vi "StageTest2.vi"() -> ()   [LabVIEW 2020]
uses:
  SettingCtrlOptions.ctl
  StageOptions.ctl
  PosCtrlOptions.ctl
  libximc.lvlib
panel:
  in  "Mode":enum16{"Raster", "Serpentine"}(ring)
  in  "Stop":bool
  in  "Y End":sgl=8.0
  in  "Y Start":sgl
  in  "X End":sgl=10.0
  in  "X Start":sgl
  in  "Pixel Count":i32=6
  out "Stage Position":cluster{sgl[], sgl[]}(graph)
  in  "Line Count":i32=6
  out "IDs":i32[](array[numeric])
  out "Calibration":cluster{dbl, "MicrostepMode":u32}[](array[cluster])
  in  "Speed (mm/s)":sgl
  out "Step Sizes(mm)":sgl[](array[numeric])
  in  "numSteps = 1mm 2":i32=100
  in  "Correction Table Path (Hidden)":path
  out "Serial nos":u32[](array[numeric])
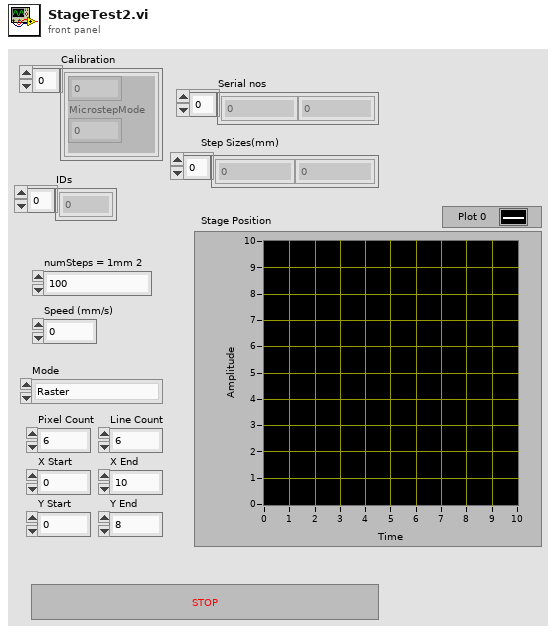
[diagram p1: front panel]
types:
  T1 = typedef "StageOptions.ctl" = enum16{"Idle", "MoveNext", "Stop Motion", "Get Pos"}
  T2 = typedef "SettingCtrlOptions.ctl" = enum16{"Set X", "Set Y", "Set X and Y", "Get Settings", "None"}
  T3 = typedef "PosCtrlOptions.ctl" = enum16{"Move X", "Move Y", "Both X and Y", "Read Pos", "None"}
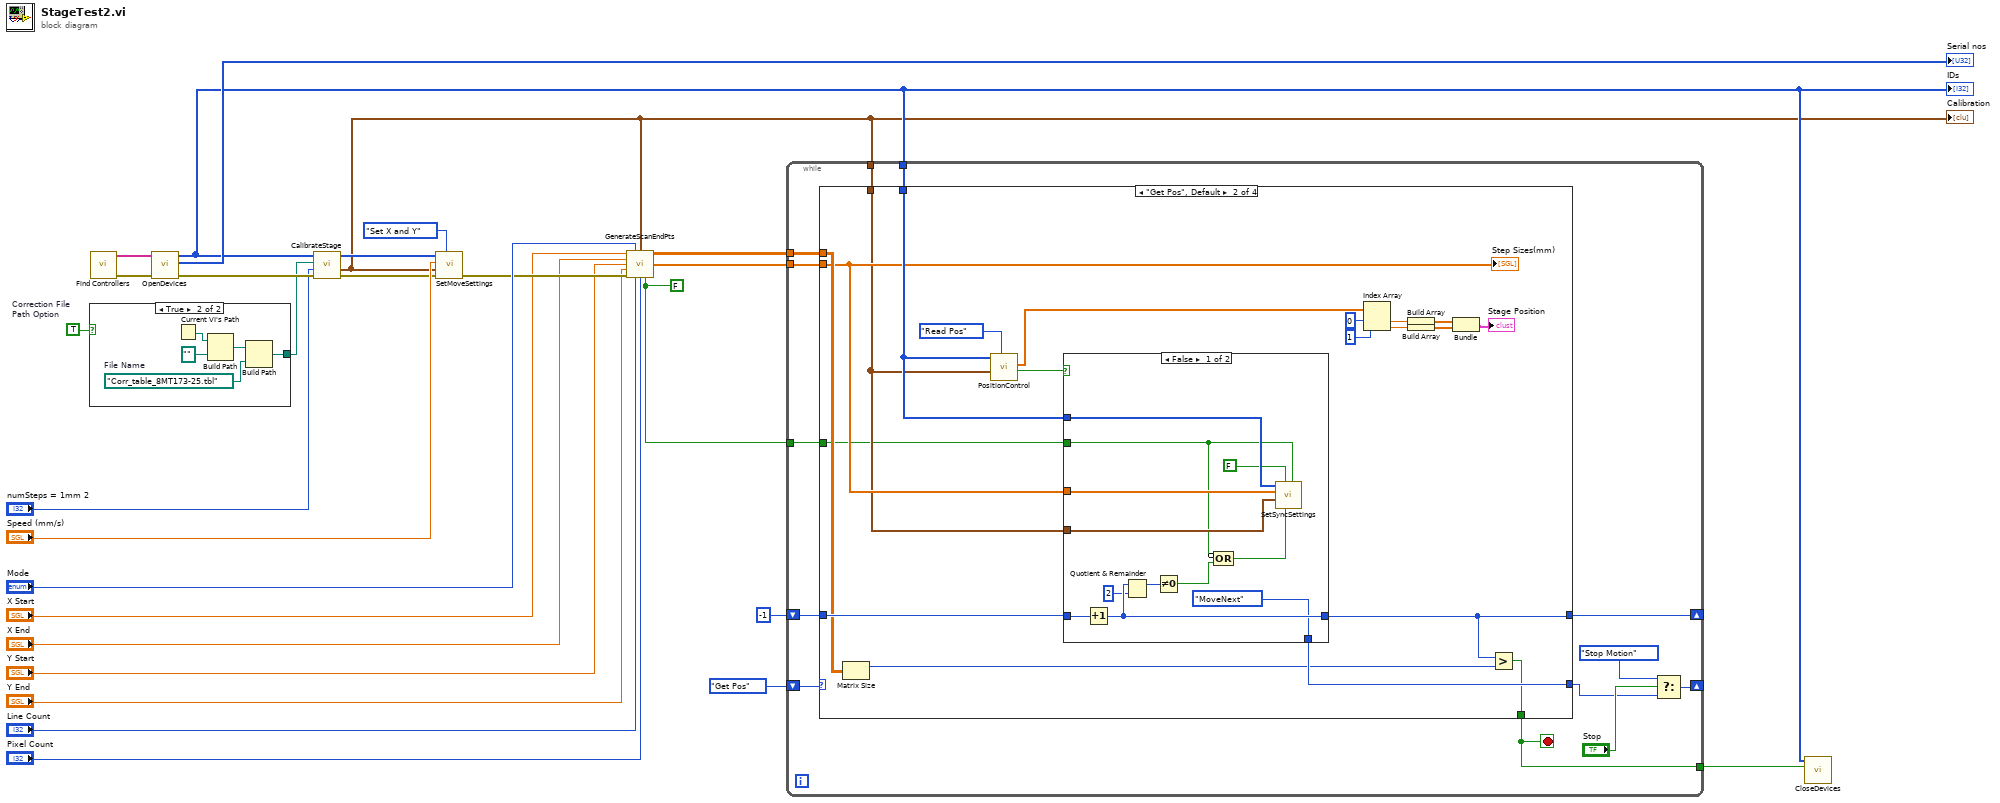
[diagram p0: block diagram]
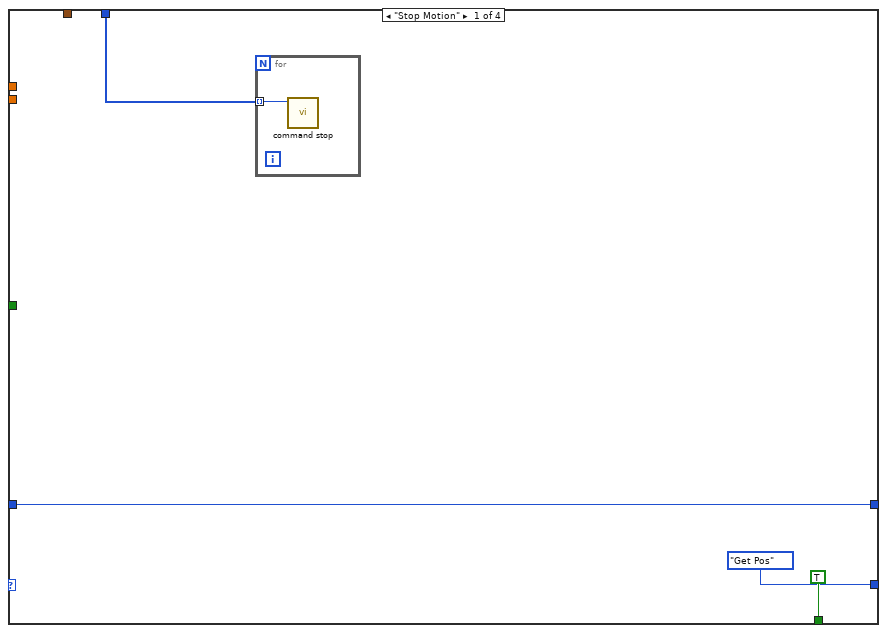
[diagram p2: hidden frame]
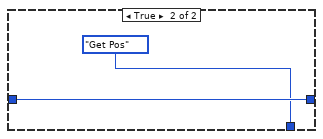
[diagram p3: hidden frame]
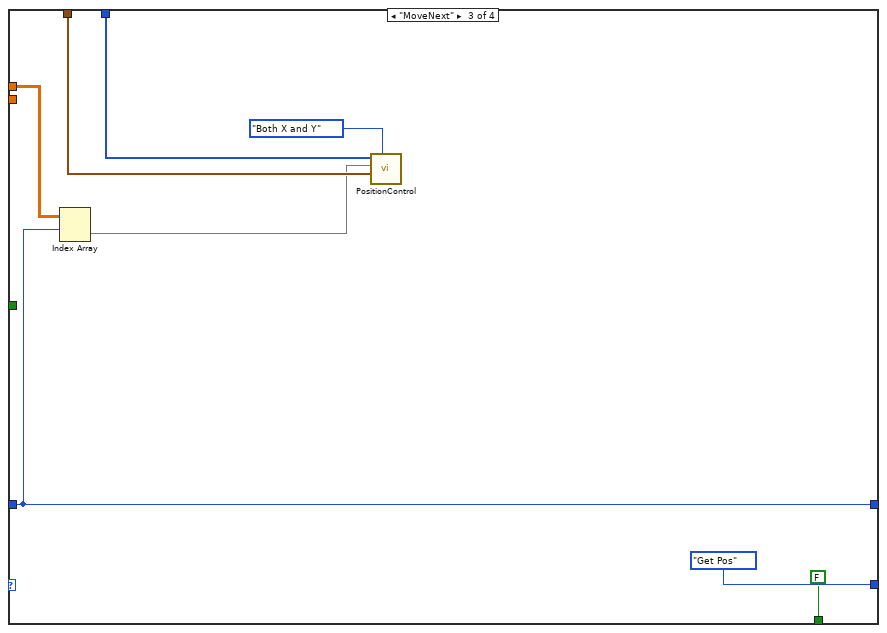
[diagram p4: hidden frame]
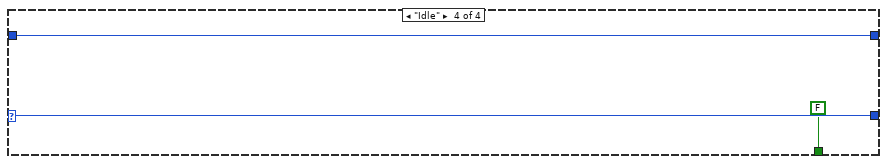
[diagram p5: hidden frame]
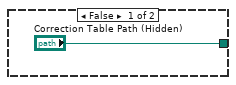
[diagram p6: hidden frame]
diagram:
  w1 = FALSE ("EdgePt/nPixelMap")
  w23 = TRUE  # Correction File Path Option
  n1 = case shown="True" w23 {
    tunnel: ["Correction Table Path (Hidden)" w29] -> w22
    frame False {
    }
    frame True {
      w30 = path "Corr_table_8MT173-25.tbl"  # File Name
      n2 = Current VI's Path() -> (path=w32:path)
      n3 = Build Path(base path=w32, name or relative path=path "") -> (appended path=w31:path)
      n4 = Build Path(base path=w31, name or relative path=w30) -> (appended path=w29:path)
    }
  }
  n5 = call "Find Controllers.vi"() -> ("error out"=w26:errorcluster, "Names"=w27:string[])  [unwired: 9 in, 1 out]
  n6 = call "OpenDevices.vi"("error In"=w26, "Names"=w27) -> ("error out"=w25:errorcluster, "Serial nos"=→"Serial nos":u32[], "IDs"=w4:i32[])  [unwired: 6 in]
  "IDs" <- w4
  n7 = call "CalibrateStage.vi"("error in (no error)"=w25, "numSteps = 1mm"="numSteps = 1mm 2", "Correction Table Path"=w22, "IDs"=w4) -> ("error out"=w6:errorcluster, "Calibration"=w2:cluster{dbl, "MicrostepMode":u32}[], "IDs Out"=w5:i32[])  [unwired: 2 in, 3 out]
  "Calibration" <- w2
  n8 = call "SetMoveSettings.vi"("Mode"=SettingCtrlOptions."Set X and Y", "error in (no error)"=w6, "Calibration"=w2, "Speed"="Speed (mm/s)", "IDs"=w5) -> ("error out"=w17:errorcluster)  [unwired: 4 in, 2 out]
  n9 = call "GenerateScanEndPts.vi"("X Start"="X Start", "Mode"="Mode", "Calibration In"=w2, "X End"="X End", "Y Start"="Y Start", "Y End"="Y End", "error in"=w17, "Line Count"="Line Count", "Pixel Count"="Pixel Count", "EdgePt/nPixelMap"=w1) -> ("Coordinate Array"=w15:sgl[][], "Step Sizes"=w8:sgl[])  [unwired: 3 in, 1 out]
  n10 = while {
    tunnel: w4 -> [w41]
    tunnel: w2 -> [w46]
    shift-right: [w37] -> _
    shift-left: StageOptions."Get Pos" -> [w45]
    tunnel: w15 -> [w44]
    shift-right: [w38] -> _
    shift-left: -1 ("index (row)") -> [w43]
    tunnel: w8 -> [w42]
    tunnel: [w40] -> w3
    tunnel: w1 -> [w34]
    stop <- w40 stop-if-true
    n11 = case shown="\"Get Pos\", Default" w45 {
      selector: w45 -> [_ _ _ w95]
      tunnel: w41 -> [w47 w55 w93 _]
      tunnel: w46 -> [_ w53 w92 _]
      tunnel: [StageOptions."Get Pos" w60 StageOptions."Get Pos" w95] -> w36
      tunnel: w44 -> [_ w59 w91 _]
      tunnel: w43 -> [w48 w62 w88 w96]
      tunnel: [w48 w57 w88 w96] -> w38
      tunnel: [TRUE w56 FALSE FALSE] -> w40
      tunnel: w42 -> [_ w54 _ _]
      tunnel: w34 -> [_ w52 _ _]
      frame "Stop Motion" {
        n12 = for {
          tunnel: w47 -> [w51] mode=indexing
          n13 = call "command stop.vi"("id"=w51) -> ()  [unwired: 9 in, 2 out]
        }
      }
      frame "Get Pos", Default {
        n14 = Matrix Size(0:w59) -> (1:w58:i32)  [unwired: 1 out]
        n15 = call "PositionControl.vi"("Mode"=PosCtrlOptions."Read Pos", "Calibration"=w53, "IDs"=w55) -> ("Moving?"=w61:bool, "Position"=w71:sgl[])  [unwired: 5 in, 2 out]
        n16 = case shown="False" w61 {
          tunnel: w62 -> [w83 w85]
          tunnel: [w82 w85] -> w57
          tunnel: [StageOptions."MoveNext" StageOptions."Get Pos"] -> w60
          tunnel: w55 -> [w80 _]
          tunnel: w54 -> [w77 _]
          tunnel: w53 -> [w79 _]
          tunnel: w52 -> [w74 _]
          frame False {
            n17 = Increment(x=w83) -> (x+1=w82:i32)
            n18 = Quotient & Remainder(x=w82, y=2) -> (x-y*floor(x/y)=w78:i32)  [unwired: 1 out]
            n19 = Not Equal To 0?(x=w78) -> (x != 0?=w73:bool)
            n20 = Compound Arithmetic op=OR(invert w74, w73) -> (w72:bool)
            n21 = call "SetSyncSettings.vi"("Periodic/nPointScan"=w74, "X SyncOut Enabled"=w72, "Y SyncOut Enabled"=FALSE, "Calibration"=w79, "Step Sizes(mm)"=w77, "IDs"=w80) -> ()  [unwired: 4 in, 2 out]
          }
          frame True {
          }
        }
        n22 = Index Array(array=w71, index #1=0 ("index"), index #2=1 ("index")) -> (element #1=w67:sgl, element #2=w66:sgl)
        n23 = Build Array(w67) -> (w69:sgl[])
        n24 = Build Array(w66) -> (w70:sgl[])
        n25 = Bundle(w69, w70) -> (→"Stage Position":cluster{sgl[], sgl[]})  [unwired: 1 in]
        n26 = Greater?(x=w57, y=w58) -> (0:w56:bool)
        "Step Sizes(mm)" <- w54
      }
      frame "MoveNext" {
        n27 = Index Array(array=w91, index (row)=w88) -> (element=w90:sgl[])  [unwired: 1 in]
        n28 = call "PositionControl.vi"("Mode"=PosCtrlOptions."Both X and Y", "Calibration"=w92, "Move to"=w90, "IDs"=w93) -> ()  [unwired: 4 in, 4 out]
      }
      frame "Idle" {
      }
    }
    n29 = Select(t=StageOptions."Stop Motion", s="Stop", f=w36) -> (s? t:f=w37:T1)
  }
  n30 = call "CloseDevices.vi"("Close"=w3, "Ids"=w4) -> ()  [unwired: 9 in, 1 out]
